vi "test1.vi"() -> ()   [LabVIEW 2015]
panel:
  out "output array":dbl[](array[numeric])
  in  "array":dbl[][](array[numeric])
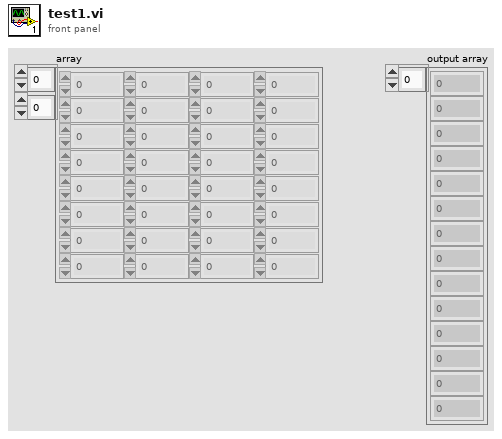
[diagram p1: front panel]
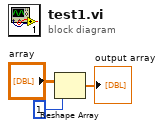
[diagram p0: block diagram]
diagram:
  n1 = Reshape Array("array", 1 ("dimension size")) -> (→"output array":dbl[])
